vi "fpga_status.vi"(8 "error in (no error)":errorcluster, 11 "5785_3.2GHz_one channel in":refnum<class "5785_3.2GHz_one channel.lvclass">) -> (0 "error out":errorcluster, 2 "pulse TX status":T1, 3 "5785_3.2GHz_one channel out":refnum<class "5785_3.2GHz_one channel.lvclass">)   [LabVIEW 2021, in "5785_3.2GHz_one channel.lvclass"]
uses:
  5785_3.2GHz_one channel.lvclass
  5785_3.2GHz_one channel.lvclass/5785_3.2GHz_one channel.ctl
  <vilib>/rvi/interface/nirviReadWriteControl/nirviReadWriteControl.xnode
  NiFpgaLv.dll
  <vilib>/Utility/error.llb/Error Cluster From Error Code.vi
  <vilib>/rvi/interface/Simulation/niFpgaSimulationCallBeginRW.vi
  <vilib>/rvi/errors/niLvFpgaAdjustHostInterfaceError.vi
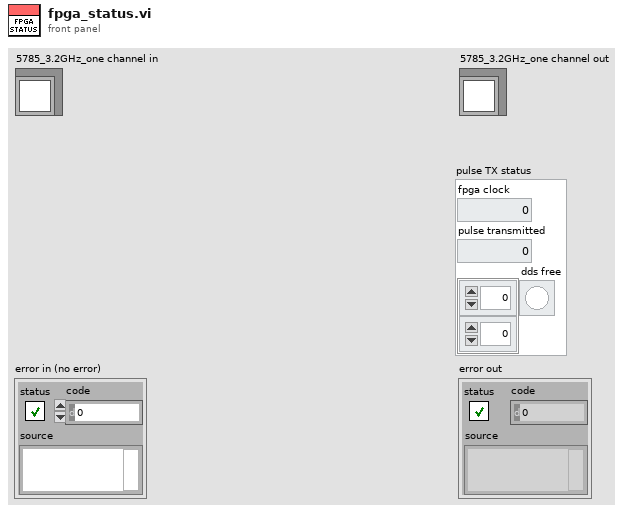
[diagram p1: front panel]
types:
  T1 = cluster{"fpga clock":dbl, "pulse transmitted":u32, "dds free":bool[][]}
  T2 = cluster{"fpga clock":u64, "pulse transmitted":u32, "dds free":bool[][]}
  T3 = cluster{"fpga clock":u64, "pulse transmitted":u32, "dds free":bool[]}
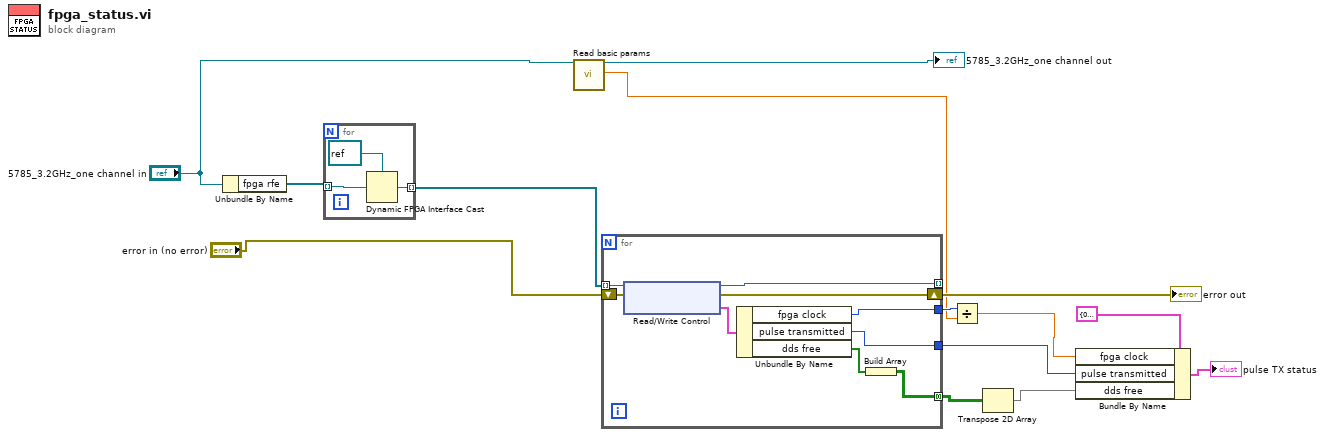
[diagram p0: block diagram]
diagram:
  n1 = Unbundle By Name("5785_3.2GHz_one channel in") -> ("fpga rfe"=w12:refnum<k20>[])
  n2 = for {
    tunnel: w12 -> [w17] mode=indexing
    tunnel: [w16] -> w13 mode=indexing
    n3 = Dynamic FPGA Interface Cast(Session In=refnum<k20> refnum ("FPGA VI Reference Out"), Type=w17) -> (Session Out=w16:refnum<k20>)
  }
  n4 = call-dynamic "Read basic params.vi"("device_type in"="5785_3.2GHz_one channel in") -> ("device_type out"=→"5785_3.2GHz_one channel out":refnum<class "5785_3.2GHz_one channel.lvclass">, "Fs  FPGA"=w1:dbl)  [unwired: 13 in, 4 out]
  n5 = for {
    tunnel: w13 -> [w23] mode=indexing
    shift-right: [w25] -> w9
    shift-left: "error in (no error)" -> [w26]
    tunnel: [w24] -> _ mode=indexing
    tunnel: [w22] -> w11 mode=concatenating
    tunnel: [w19] -> w8
    tunnel: [w20] -> w14
    n6 = xnode "Read/Write Control"("FPGA VI Reference In"=w23, "error in"=w26) -> ("FPGA VI Reference Out"=w24:refnum<k20>, "error out"=w25:errorcluster, "pulse TX status"=w21:T3)
    n7 = Unbundle By Name(w21) -> ("fpga clock"=w20:u64, "pulse transmitted"=w19:u32, "dds free"=w18:bool[])
    n8 = Build Array(w18) -> (w22:bool[][])
  }
  "error out" <- w9
  n9 = Divide(x=w14, y=w1) -> (x/y=w7:dbl)
  n10 = Transpose 2D Array(2D array=w11) -> (transposed array=w4:bool[][])
  n11 = Bundle By Name(cluster=T2 {"fpga clock"=0, "pulse transmitted"=0, "dds free"=[[FALSE, FALSE, FALSE, FALSE, FALSE, FALSE, FALSE, FALSE, FALSE, FALSE, FALSE, FALSE, FALSE, FALSE, FALSE, FALSE]]} ("pulse TX status"), "fpga clock"=w7, "pulse transmitted"=w8, "dds free"=w4) -> (→"pulse TX status":T2)
